vi "Change Address.vi"(8 "Error In (No Error)":errorcluster, 9 "New Address In":string="b", 10 "Sensor Address In":string="a", 11 "RS232 Port In":refnum<visa-resource-name>) -> (0 "Error Out":errorcluster, 1 "Success?":bool, 3 "RS232 Port Out":refnum<visa-resource-name>)   [LabVIEW 2015, in "SDI-12.lvlib"]
doc: "Changes the address of a sensor.\n\naAb!\n\na = Current Address\nA = Address Change Command\nb = New Address"
uses:
  SDI-12.lvlib
panel:
  out "Sensor Address Out":string="a"
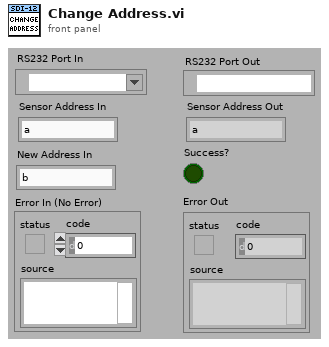
[diagram p1: front panel]
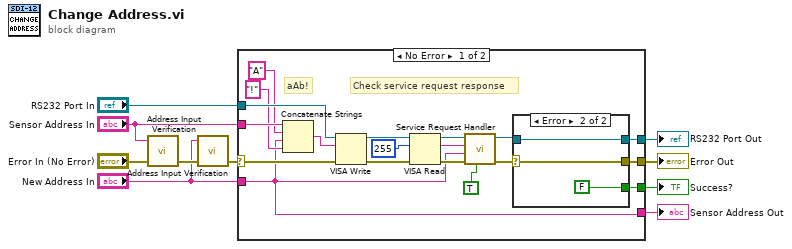
[diagram p0: block diagram]
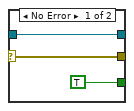
[diagram p2: hidden frame]
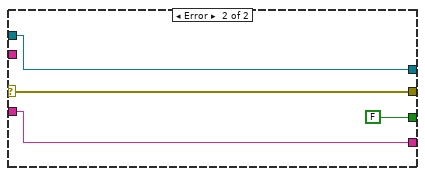
[diagram p3: hidden frame]
diagram:
  n1 = call "Address Input Verification.vi"("Error In (No Error)"="Error In (No Error)", "Sensor Address In (a)"="Sensor Address In") -> ("Error Out"=w5:errorcluster)  [unwired: 2 in, 1 out]
  n2 = call "Address Input Verification.vi"("Error In (No Error)"=w5, "Sensor Address In (a)"="New Address In") -> ("Error Out"=w4:errorcluster)  [unwired: 2 in, 1 out]
  n3 = case shown="No Error" w4 {
    selector: w4 -> [w27 w38]
    tunnel: [w26 FALSE ("sensor response?")] -> w10
    tunnel: [w23 w38] -> w9
    tunnel: "RS232 Port In" -> [w22 w37]
    tunnel: "Sensor Address In" -> [w21 _]
    tunnel: "New Address In" -> [w15 w36]
    tunnel: [w17 w37] -> w2
    tunnel: [w15 w36] -> w1
    frame No Error {
      # "aAb!"
      # "Check service request response"
      n4 = Concatenate Strings(w21, "A" ("string"), w15, "!" ("string")) -> (w18:string)
      n5 = VISA Write(VISA resource name=w22, write buffer=w18, error in (no error)=w27) -> (VISA resource name out=w14:refnum<visa-resource-name>, error out=w13:errorcluster)  [unwired: 1 out]
      n6 = VISA Read(VISA resource name=w14, byte count=u32 255, error in (no error)=w13) -> (VISA resource name out=w25:refnum<visa-resource-name>, read buffer=w24:string, error out=w28:errorcluster)  [unwired: 1 out]
      n7 = call "Service Request Handler.vi"("Check address? (False)"=TRUE ("Check address? (false)"), "Error In (No Error)"=w28, "Expected Sensor Address (a)"=w15, "Service Request"=w24, "RS232 Port In"=w25) -> ("Error Out"=w11:errorcluster, "RS232 Port Out"=w12:refnum<visa-resource-name>)  [unwired: 3 in, 2 out]
      n8 = case shown="Error" w11 {
        selector: w11 -> [w32 w33]
        tunnel: [w32 w33] -> w23
        tunnel: w12 -> [w31 w35]
        tunnel: [w31 w35] -> w17
        tunnel: [TRUE ("sensor response?") FALSE ("sensor response?")] -> w26
        frame No Error {
        }
        frame Error {
        }
      }
    }
    frame Error {
    }
  }
  "Error Out" <- w9
  "Success?" <- w10
  "Sensor Address Out" <- w1
  "RS232 Port Out" <- w2
